vi "Create.vi"(5 "XY Position":refnum<vi>, 7 "Z Position":refnum<vi>, 8 "error in (no error)":errorcluster) -> (0 "error out":errorcluster, 3 "Gantry Status out":refnum<class "Gantry Status.lvclass">)   [LabVIEW 2011, in "Gantry Status.lvclass"]
uses:
  Gantry Status.lvclass
  Gantry Status.lvclass/Gantry Status.ctl
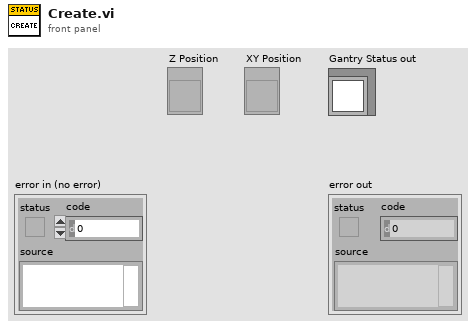
[diagram p1: front panel]
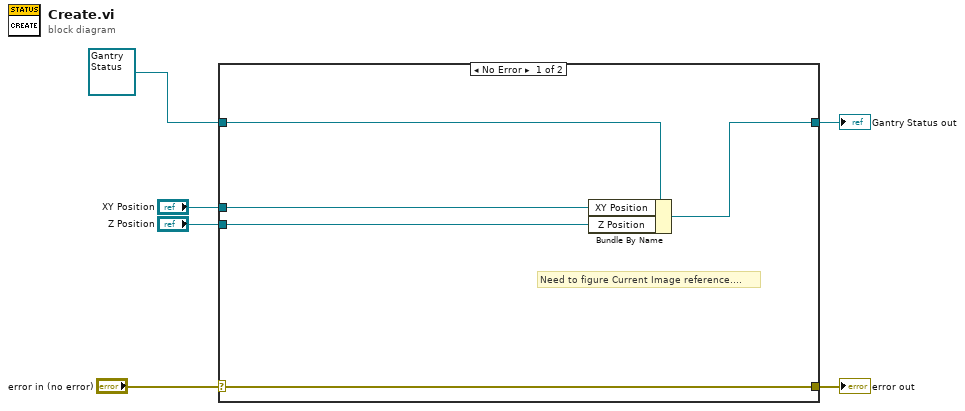
[diagram p0: block diagram]
diagram:
  n1 = case shown="No Error" "error in (no error)" {
    selector: "error in (no error)" -> [w11 w13]
    tunnel: [w11 w13] -> w5
    tunnel: [w9 w12] -> w3
    tunnel: refnum<class "Gantry Status.lvclass"> refnum ("Gantry Status in") -> [w10 w12]
    tunnel: "XY Position" -> [w8 _]
    tunnel: "Z Position" -> [w7 _]
    frame No Error {
      # "Need to figure Current Image reference...."
      n2 = Bundle By Name(cluster=w10, "XY Position"=w8, "Z Position"=w7) -> (w9:refnum<class "Gantry Status.lvclass">)
    }
    frame Error {
    }
  }
  "error out" <- w5
  "Gantry Status out" <- w3
